vi "Globals.vi"() -> ()   [LabVIEW 2015]
panel:
  in  "block_ch":u8=1
  in  "LED off":bool
  in  "vfreq":u8=3
  in  "area_lines_binning":u32=3
  in  "region_size":u8[](array[numeric])
  in  "BlockSyncStart":bool=TRUE
  in  "use GPX":bool=TRUE
  in  "GPX Offset":u32=3
  in  "nor":u32=1100
  in  "mshut":bool
  in  "lines":u32=3
  in  "showOnePixelGraph":bool=TRUE
  in  "CoolCam":bool=TRUE
  in  "board_sel_offset":u32=3
  in  "cam gain":u32=3
  in  "maddr of IOCTRL":u8=2
  in  "debug_mode":bool=TRUE
  in  "use DAC":bool=TRUE
  in  "maddr of ADC":u8=1
  in  "camera system select":u8=2
  in  "CAMCNT":u32=2
  in  "maddr of CAM":u8
  in  "cam_sel":u8
  in  "nosnobchanged":bool
  in  "board_sel":u32=3
  in  "nob":u32=4
  in  "dioden 2":u16[][](array[numeric])
  in  "dioden 1":u16[][](array[numeric])
  in  "stime_in_ms":dbl=0.1
  in  "nos":u32=1100
  in  "PIXEL":u32=1088
  in  "boards":u32=1
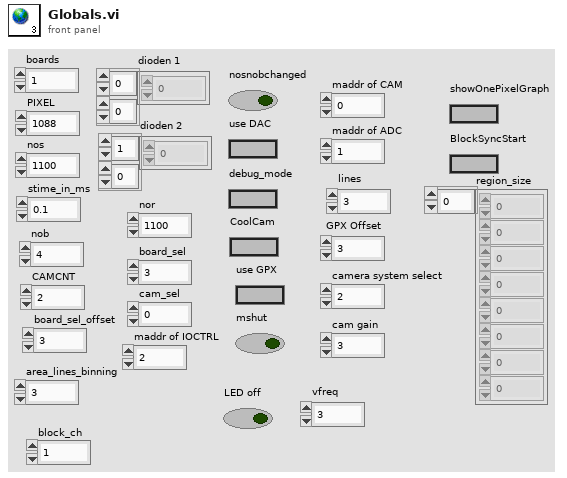
[diagram p1: front panel]
diagram:
